vi "HGF_ThreadTask.appendData2Variant.vi"(0 "initData":variant, 2 "taskTrigger":refnum<class "HGF_Event.lvclass">, 3 "taskDestination":refnum<class "HGF_Event.lvclass">, 4 "objectArray":refnum<class>[](array[class]), 5 "error in (no error)":errorcluster, 7 "exceptionEvent":refnum<class "HGF_TriggeredEvent.lvclass">) -> (14 "dup initData":variant, 19 "error out":errorcluster)   [LabVIEW 2014, in "HGF_BaseClasses.lvlib" / "HGF_ThreadTask.lvclass"]
doc: "Append initialize data to variant."
uses:
  HGF_ThreadTask.lvclass
  HGF_Event/HGF_Event.lvclass
  HGF_TriggeredEvent/HGF_TriggeredEvent.lvclass
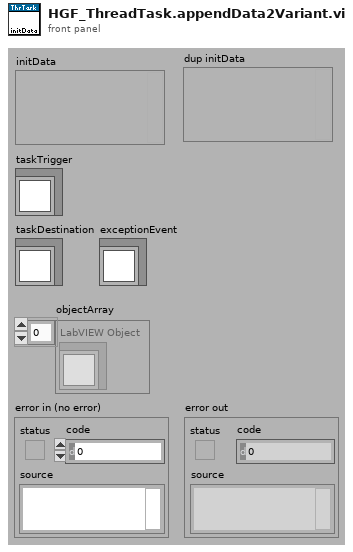
[diagram p1: front panel]
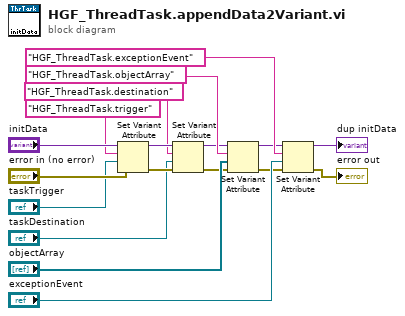
[diagram p0: block diagram]
diagram:
  n1 = Set Variant Attribute(Variant="initData", name="HGF_ThreadTask.trigger", value="taskTrigger", error in="error in (no error)") -> (Variant out=w14:variant, error out=w13:errorcluster)  [unwired: 1 out]
  n2 = Set Variant Attribute(Variant=w14, name="HGF_ThreadTask.destination", value="taskDestination", error in=w13) -> (Variant out=w7:variant, error out=w8:errorcluster)  [unwired: 1 out]
  n3 = Set Variant Attribute(Variant=w7, name="HGF_ThreadTask.objectArray", value="objectArray", error in=w8) -> (Variant out=w4:variant, error out=w2:errorcluster)  [unwired: 1 out]
  n4 = Set Variant Attribute(Variant=w4, name="HGF_ThreadTask.exceptionEvent", value="exceptionEvent", error in=w2) -> (Variant out=→"dup initData":variant, error out=→"error out":errorcluster)  [unwired: 1 out]
